vi "VNA Driver.vi"(5 "VNA Driver or\nVNA Configuration (\"\")":string, 6 "Drv Refnum":T2, 7 "VNA Command":T3=enum."MEASURE", 8 "error in (no error)":errorcluster, 9 "Miscellaneous Parameters":T1, 10 "VNA Stimulus":T8={"Use Instrument Settings"=FALSE, "Blank Frequencies"=FALSE, "Sweep Type"=enum."Linear", "Sweep"={"Fstart"=500.0, "Fstop"=1500.0, "Units"=enum."MHz", "Points"=201}, "Power (dBm)"=999.0, "IFBW (Hz)"=-1.0, "Sweep Time (s)"=-1.0, "Calibration"={"State"=FALSE, "String"=""}} {"Sweep Time (s)" format="%.3g"}, 11 "Parameters to Measure":T4[](array[typedef]) {"Channel" min=1 max=99 step=1; "Parameter"."Stimulus Port" min=1 step=1; "Parameter"."Response Port" min=1 step=1}) -> (0 "error out":errorcluster, 1 "VNA Flat Output":string, 2 "SP Data":T10, 3 "Parameters Measured":T4[](array[typedef]) {"Channel" min=1 max=99 step=1; "Parameter"."Stimulus Port" min=1 step=1; "Parameter"."Response Port" min=1 step=1}, 4 "dup Drv Refnum":T2)   [LabVIEW 2011]
uses:
  tests/S Parameter/TypeDefs/SP Data.ctl
  tests/S Parameter/TypeDefs/SP Stimulus Parameters.ctl
  tests/S Parameter/TypeDefs/SP Frequency Units.ctl
  tests/S Parameter/TypeDefs/SP Calibration State.ctl
  tests/S Parameter/TypeDefs/SP Parameter to Measure.ctl
  tests/S Parameter/TypeDefs/SP Parameter.ctl
  tests/S Parameter/TypeDefs/SP Measurement Format.ctl
  VNA Command.ctl
  VNA Driver Ref.ctl
  tests/S Parameter/TypeDefs/SP Miscellaneous Parameters.ctl
panel:
  in  "DEBUG?":bool
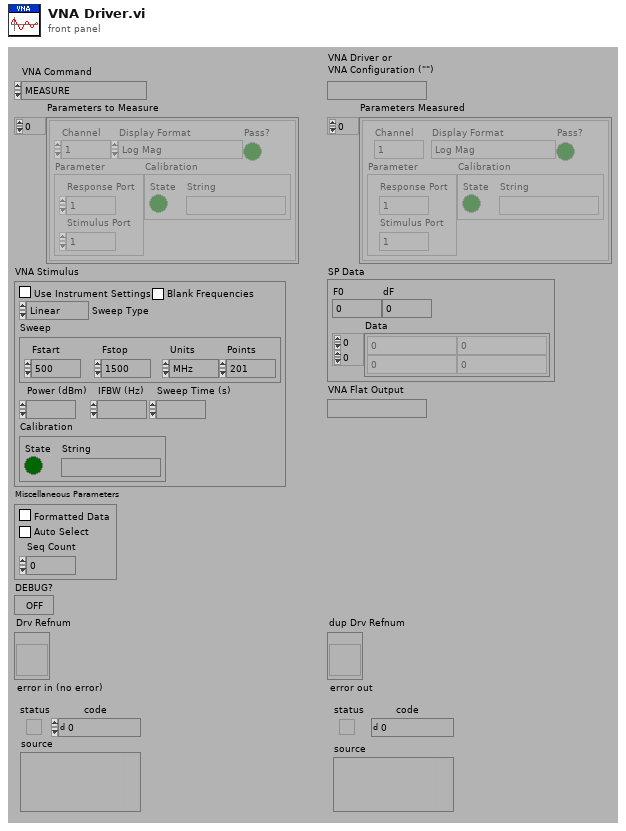
[diagram p1: front panel]
types:
  T1 = typedef "SP Miscellaneous Parameters.ctl" = cluster{"Formatted Data":bool, "Auto Select":bool, "Seq Count":u32}
  T2 = typedef "VNA Driver Ref.ctl" = refnum<vi>
  T3 = typedef "VNA Command.ctl" = enum16{"LOAD", "INITIALIZE", "PRESET", "GET STIMULUS", "SET STIMULUS", "GET CALIBRATION", "CALIBRATE", "RESTORE", "MEASURE", "RELEASE", "UNLOAD", "CONFIRM", "SORT"}
  T4 = typedef "SP Parameter to Measure.ctl" = cluster{"Channel":i8, "Parameter":T5, "Calibration":T6, "Display Format":T7, "Pass?":bool}
  T5 = typedef "SP Parameter.ctl" = cluster{"Stimulus Port":i8, "Response Port":i8}
  T6 = typedef "SP Calibration State.ctl" = cluster{"State":bool, "String":string}
  T7 = typedef "SP Measurement Format.ctl" = enum32{"Log Mag", "Phase", "Delay", "Smith (R+jX)", "Polar (Re/Im)", "Linear Mag", "SWR", "Real", "Imaginary", "Smith (Lin/Phase)", "Smith (Log/Phase)", "Smith (Real/Imag)", "Smith (G+jB)", "Polar (Lin/Phase)", "Polar (Log/Phase)", "Expanded Phase", "Positive Phase", "Inverted Smith", "Unwrapped Phase", "Power Out", "Power In", "Linear Mag/Phase", "Log Mag/Phase", "Real/Imaginary"}
  T8 = typedef "SP Stimulus Parameters.ctl" = cluster{"Use Instrument Settings":bool, "Blank Frequencies":bool, "Sweep Type":enum32{"Linear", "Logarithmic", "List", "Power", "CW"}, "Sweep":cluster{"Fstart":dbl, "Fstop":dbl, "Units":T9, "Points":i32}, "Power (dBm)":dbl, "IFBW (Hz)":dbl, "Sweep Time (s)":dbl, "Calibration":T6}
  T9 = typedef "SP Frequency Units.ctl" = enum16{"Hz", "kHz", "MHz", "GHz", "Points"}
  T10 = typedef "SP Data.ctl" = cluster{"F0":dbl, "dF":dbl, "Data":cdb[][]}
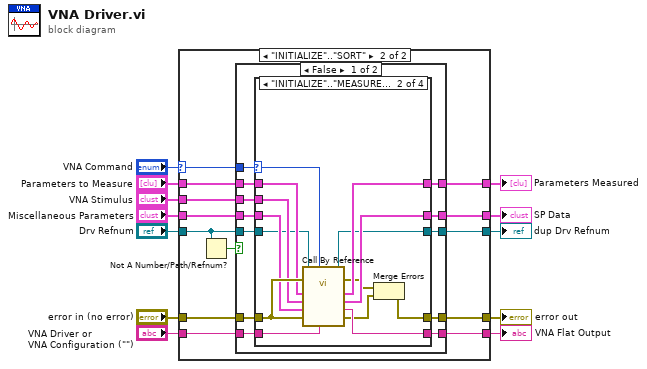
[diagram p0: block diagram]
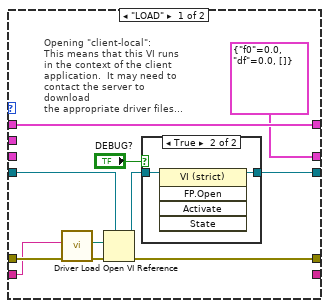
[diagram p2: hidden frame]
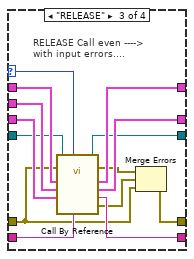
[diagram p5: hidden frame]
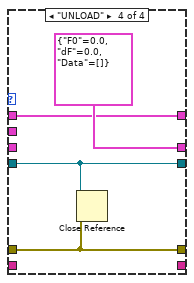
[diagram p6: hidden frame]
diagram:
  n1 = case shown="\"INITIALIZE\"..\"SORT\"" "VNA Command" {
    selector: "VNA Command" -> [_ w29]
    tunnel: "error in (no error)" -> [w23 w39]
    tunnel: "VNA Stimulus" -> [_ w38]
    tunnel: "Parameters to Measure" -> [w22 w37]
    tunnel: [w22 w36] -> w9
    tunnel: [cluster{"f0":dbl, "df":dbl, cdb[][]} {"f0"=0.0, "df"=0.0, []} ("S Parameters") w35] -> w8
    tunnel: "VNA Driver or\nVNA Configuration (\"\")" -> [w20 w34]
    tunnel: [_ w33] -> w6
    tunnel: [w19 w32] -> w5
    tunnel: "Drv Refnum" -> [w18 w28]
    tunnel: [w17 w31] -> w3
    tunnel: "Miscellaneous Parameters" -> [_ w30]
    frame "LOAD" {
      # "Opening \"client-local\":\nThis means that this VI runs\nin the context of the client\napplication.  It may need to\ncontact the server to download\nthe appropriate driver files..."
      n2 = call "Driver Load.vi"("error in (no error)"=w23, "DriverID DriverType (\"\")"=w20) -> ("error out"=w15:errorcluster, "Driver Component Path"=w14:path)  [unwired: 1 in, 7 out]
      n3 = Open VI Reference(type specifier VI Refnum (for type only)=w18, vi path=w14, error in (no error)=w15) -> (vi reference=w13:T2, error out=w17:errorcluster)  [unwired: 3 out]
      n4 = case shown="True" "DEBUG?" {
        tunnel: w13 -> [w24 w26]
        tunnel: [w24 w25] -> w19
        frame False {
        }
        frame True {
          n5 = invoke class="VI (strict)" method="FP.Open"(reference=w26) -> (reference out=w25:T2)  [unwired: 4 in, 4 out]
        }
      }
    }
    frame "INITIALIZE".."SORT" {
      n6 = Not A Number/Path/Refnum?(number/path/refnum=w28) -> (NaN/Path/Refnum?=w27:bool)
      n7 = case shown="False" w27 {
        tunnel: w39 -> [w51 w89]
        tunnel: w38 -> [w50 _]
        tunnel: w37 -> [w49 w91]
        tunnel: [w48 w91] -> w36
        tunnel: [w47 _] -> w35
        tunnel: w34 -> [w46 w88]
        tunnel: [w45 w88] -> w33
        tunnel: [w44 w90] -> w32
        tunnel: w28 -> [w43 w90]
        tunnel: [w42 w89] -> w31
        tunnel: w30 -> [w41 _]
        tunnel: w29 -> [w40 _]
        frame False {
          n8 = case shown="\"INITIALIZE\"..\"MEASURE\", \"CONFIRM\", \"SORT\"" w40 {
            selector: w40 -> [_ w62 w77 _]
            tunnel: w51 -> [w55 w68 w70 w85]
            tunnel: w50 -> [_ w63 w78 _]
            tunnel: w49 -> [w52 w65 w80 w84]
            tunnel: [w52 w66 w81 w84] -> w48
            tunnel: [_ w67 w82 T10 {"F0"=0.0, "dF"=0.0, "Data"=[]} ("S Parameters")] -> w47
            tunnel: [w55 w69 w83 w85] -> w42
            tunnel: w46 -> [w54 w61 w76 _]
            tunnel: [w54 w64 w79 _] -> w45
            tunnel: [w53 w56 w71 w86] -> w44
            tunnel: w43 -> [w53 w57 w72 w86]
            tunnel: w41 -> [_ w60 w75 _]
            frame "LOAD" {
              # "This will not ever run."
            }
            frame "INITIALIZE".."MEASURE", "CONFIRM", "SORT" {
              n9 = call-by-ref "?"(reference=w57, error in=w68, "VNA Configuration (\"\")"=w61, "VNA Command"=w62, "error in (no error)"=w68, "Miscellaneous Parameters"=w60, "VNA Stimulus"=w63, "Parameters to Measure"=w65) -> (reference out=w56:T2, error out=w58:errorcluster, 0:"error out"=w59:errorcluster, "VNA Flat Output"=w64:string, "VNA Measurements"=w67:T10, "Parameters Measured"=w66:T4[])  [unwired: 2 in]
              n10 = Merge Errors(w58, w59) -> (w69:errorcluster)
            }
            frame "RELEASE" {
              # "RELEASE Call even ---->\nwith input errors...."
              n11 = call-by-ref "?"(reference=w72, error in=w70, "VNA Configuration (\"\")"=w76, "VNA Command"=w77, "Miscellaneous Parameters"=w75, "VNA Stimulus"=w78, "Parameters to Measure"=w80) -> (reference out=w71:T2, error out=w73:errorcluster, 0:"error out"=w74:errorcluster, "VNA Flat Output"=w79:string, "VNA Measurements"=w82:T10, "Parameters Measured"=w81:T4[])  [unwired: 3 in]
              n12 = Merge Errors(w73, w74, w70) -> (w83:errorcluster)
            }
            frame "UNLOAD" {
              n13 = Close Reference(reference=w86, error in (no error)=w85) -> ()  [unwired: 1 out]
            }
          }
        }
        frame True {
          # "If the reference is not valid\nno operation is performed."
        }
      }
    }
  }
  "error out" <- w3
  "SP Data" <- w8
  "Parameters Measured" <- w9
  "VNA Flat Output" <- w6
  "dup Drv Refnum" <- w5
